vi "FFT Buffer Manager.vi"(6 "FFT Samples":i32=50000, 7 "Function":T1, 8 "error in":errorcluster, 9 "Unique Channel Identifier":string, 10 "Waveform":waveform(dbl), 11 "Plugin in":refnum<class "FFT.lvclass">) -> (0 "error out":errorcluster, 1 "Data Valid":bool, 2 "Data":dbl[](array[numeric]), 3 "Plugin out":refnum<class "FFT.lvclass">)   [LabVIEW 2024, in "FFT.lvlib" / "FFT.lvclass"]
uses:
  FFT.lvclass
  C:/Program Files/National Instruments/LabVIEW 2024/vi.lib/FlexLogger/SDK/PluginSDK.lvlibp/PEFClasses/SDK/Processing Element/Processing Element.lvclass
  FFT Buffer Manager Function.ctl
  <vilib>/FlexLogger/SDK/PluginSDK.lvlibp/PEFClasses/SDK/Processing Element/Read Alias.vi
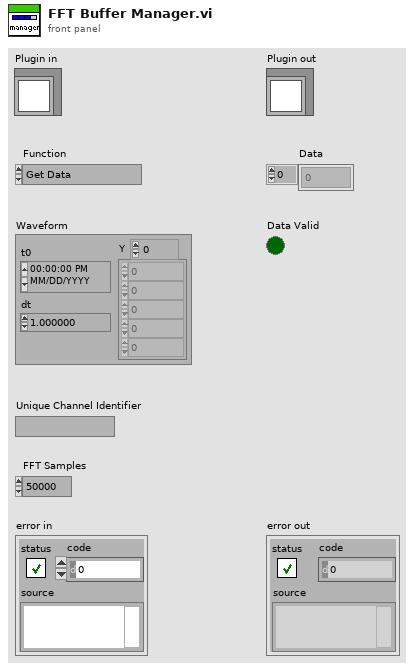
[diagram p1: front panel]
types:
  T1 = typedef "FFT.lvlib/FFT.lvclass/FFT Buffer Manager Function.ctl" = enum16{"Get Data", "Buffer Data", "Reset Data"}
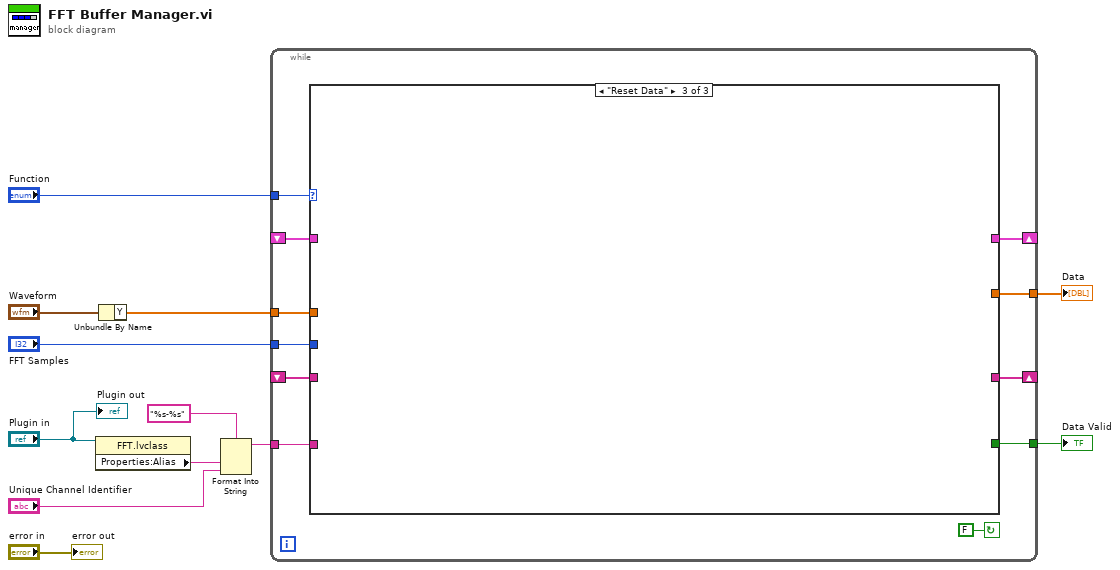
[diagram p0: block diagram]
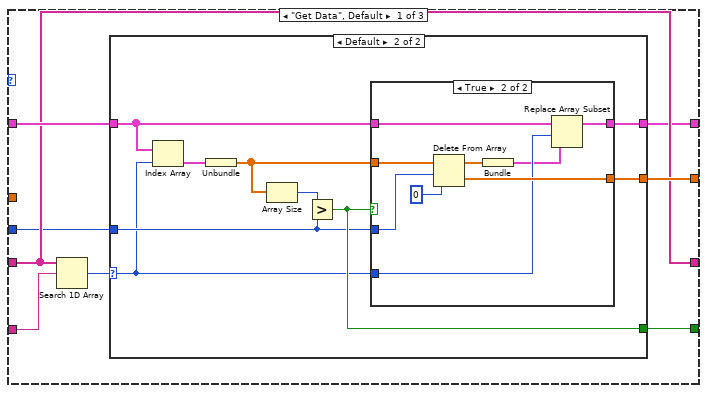
[diagram p2: hidden frame]
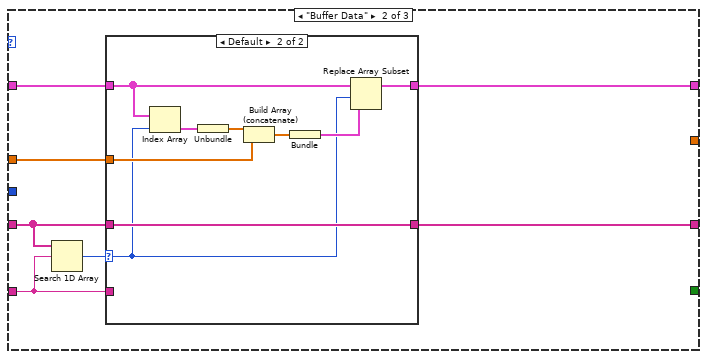
[diagram p5: hidden frame]
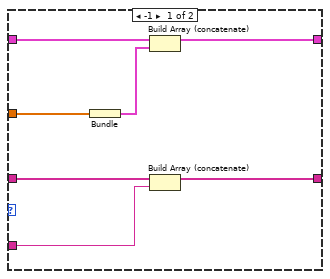
[diagram p6: hidden frame]
diagram:
  n1 = property class="FFT.lvclass"(reference="Plugin in") -> ("Properties:Alias"=w8:string)  [unwired: 1 in, 2 out]
  n2 = Unbundle By Name("Waveform") -> ("Y"=w4:dbl[])
  n3 = Format Into String(format string="%s-%s", w8, "Unique Channel Identifier") -> (resulting string=w7:string)  [unwired: 2 in, 1 out]
  n4 = while {
    tunnel: "Function" -> [w23]
    shift-right: [w16] -> _
    shift-left: _ -> [w22]
    shift-right: [w15] -> _
    shift-left: _ -> [w19]
    tunnel: w7 -> [w21]
    tunnel: [w20] -> w5
    tunnel: [w18] -> w3
    tunnel: w4 -> [w17]
    tunnel: "FFT Samples" -> [w13]
    stop <- FALSE continue-if-true
    n5 = case shown="\"Reset Data\"" w23 {
      tunnel: w22 -> [w26 w56 _]
      tunnel: w21 -> [w31 w55 _]
      tunnel: [w29 _ _] -> w20
      tunnel: w19 -> [w27 w57 _]
      tunnel: [w28 _ _] -> w18
      tunnel: w17 -> [_ w52 _]
      tunnel: [w26 w54 _] -> w16
      tunnel: [w25 w53 _] -> w15
      tunnel: w13 -> [w24 _ _]
      frame "Get Data", Default {
        n6 = Search 1D Array(1D array=w26, element=w31) -> (index of element=w30:i32)  [unwired: 1 in]
        n7 = case shown="Default" w30 {
          selector: w30 -> [_ w35]
          tunnel: [_ w39] -> w29
          tunnel: w27 -> [w32 w34]
          tunnel: w24 -> [_ w37]
          tunnel: [_ w36] -> w28
          tunnel: [w32 w33] -> w25
          frame -1 {
          }
          frame Default {
            n8 = Index Array(array=w34, index=w35) -> (element=w41:cluster{"Y":dbl[]})
            n9 = Unbundle(w41) -> ("Y"=w38:dbl[])
            n10 = Array Size(array=w38) -> (size(s)=w40:i32)
            n11 = Greater?(x=w40, y=w37) -> (0:w39:bool)
            n12 = case shown="True" w39 {
              tunnel: w38 -> [_ w50]
              tunnel: w37 -> [_ w49]
              tunnel: [_ w51] -> w36
              tunnel: w35 -> [_ w46]
              tunnel: w34 -> [w42 w45]
              tunnel: [w42 w43] -> w33
              frame False {
              }
              frame True {
                n13 = Delete From Array(array=w50, length=w49, index=0) -> (deleted portion=w51:dbl[], array with subset deleted=w47:dbl[])
                n14 = Bundle("Y"=w47) -> (w44:cluster{"Y":dbl[]})  [unwired: 1 in]
                n15 = Replace Array Subset(array=w45, new element=w44, index=w46) -> (w43:cluster{"Y":dbl[]}[])
              }
            }
          }
        }
      }
      frame "Buffer Data" {
        n16 = Search 1D Array(1D array=w56, element=w55) -> (index of element=w58:i32)  [unwired: 1 in]
        n17 = case shown="Default" w58 {
          selector: w58 -> [_ w66]
          tunnel: w57 -> [w62 w70]
          tunnel: w56 -> [w65 w67]
          tunnel: w55 -> [w64 _]
          tunnel: [w63 w67] -> w54
          tunnel: [w61 w68] -> w53
          tunnel: w52 -> [w60 w72]
          frame -1 {
            n18 = Bundle("Y"=w60) -> (w59:cluster{"Y":dbl[]})  [unwired: 1 in]
            n19 = Build Array (concatenate)(w62, w59) -> (w61:cluster{"Y":dbl[]}[])
            n20 = Build Array (concatenate)(w65, w64) -> (w63:string[])
          }
          frame Default {
            n21 = Index Array(array=w70, index=w66) -> (element=w74:cluster{"Y":dbl[]})
            n22 = Unbundle(w74) -> ("Y"=w73:dbl[])
            n23 = Build Array (concatenate)(w73, w72) -> (w71:dbl[])
            n24 = Bundle(w71) -> (w69:cluster{dbl[]})  [unwired: 1 in]
            n25 = Replace Array Subset(array=w70, new element=w69, index=w66) -> (w68:cluster{"Y":dbl[]}[])
          }
        }
      }
      frame "Reset Data" {
      }
    }
  }
  "Data Valid" <- w5
  "Data" <- w3
  "error out" <- "error in"
  "Plugin out" <- "Plugin in"
